vi "epoch microsecond to epoch access point.vi"(11 "epoch_micro_second":cluster{}) -> (3 "function return":u64)   [LabVIEW 2019, in "apdm.lvlib"]
doc: "APDM_EXPORT uint64_t apdm_epoch_microsecond_to_epoch_access_point(const uint64_t epoch_micro_second);"
uses:
  apdm.lvlib
  Lee Lab/CP FES Walking 2018/Code/Working/LabVIEW/apdm.dll
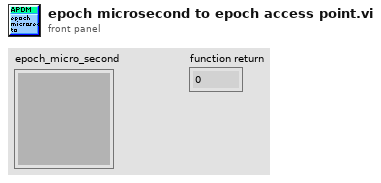
[diagram p1: front panel]
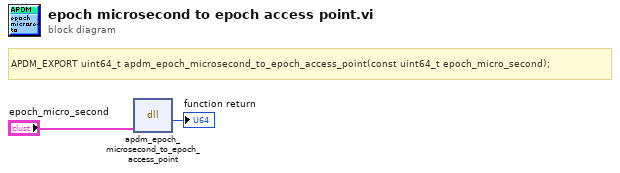
[diagram p0: block diagram]
diagram:
  # "APDM_EXPORT uint64_t apdm_epoch_microsecond_to_epoch_access_point(const uint64_t epoch_micro_second);"
  n1 = dll-call lib="C:/Users/jfalesi/Dropbox/Lee Lab/CP FES Walking 2018/Code/Working/LabVIEW/apdm.*" fn="apdm_epoch_microsecond_to_epoch_access_point"("epoch_micro_second"="epoch_micro_second") -> (→"function return":u64)  [unwired: 4 in, 2 out]
